vi "n set rot center.vi"(8 "error in (no error)":errorcluster, 9 "center_y":i32, 10 "center_x":i32, 11 "n":u16) -> (0 "error out":errorcluster)   [LabVIEW 2015, in "SCANalone4x64.lvlib"]
doc: "__declspec(dllimport) void __stdcall n_set_rot_center(unsigned short n, long center_x, long center_y);"
uses:
  <userlib>/SCANalone4x64/SCANalone4x64.lvlib
  <userlib>/SCANalone4x64/SCANalone4x64.dll
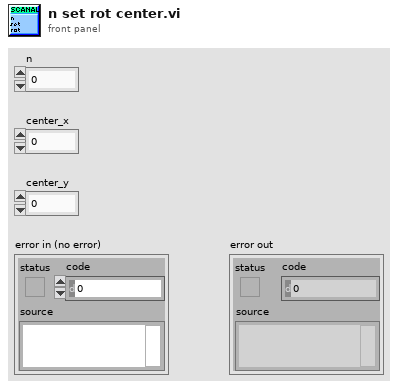
[diagram p1: front panel]
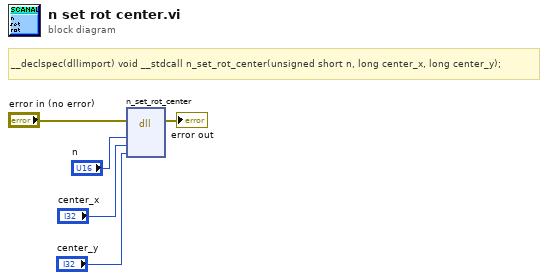
[diagram p0: block diagram]
diagram:
  # "__declspec(dllimport) void __stdcall n_set_rot_center(unsigned short n, long center_x, long center_y);"
  n1 = dll-call lib="C:/Program Files/National Instruments/LabVIEW 2015/user.lib/SCANalone4x64/SCANalone4x64.*" fn="n_set_rot_center"(error in="error in (no error)", "n"="n", "center_x"="center_x", "center_y"="center_y") -> (error out=→"error out":errorcluster)  [unwired: 6 in, 1 out]
